vi "checkMotorOverheat.vi"(8 "error in (no error)":errorcluster, 11 "Model in":refnum<class "Model.lvclass">) -> (0 "error out":errorcluster, 3 "Model out":refnum<class "Model.lvclass">)   [LabVIEW 2015]
uses:
  ApplicationElements/Thermocouple/Thermocouple.lvclass
  Model.lvclass
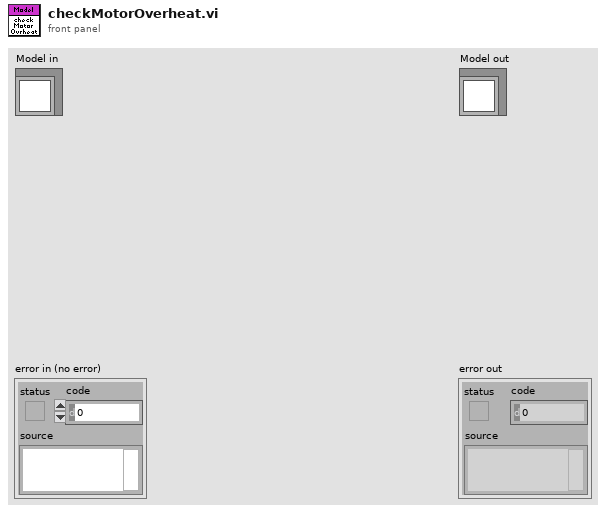
[diagram p1: front panel]
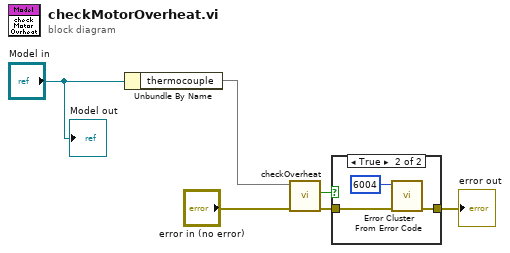
[diagram p0: block diagram]
diagram:
  n1 = Unbundle By Name("Model in") -> ("thermocouple"=w4)
  n2 = call "checkOverheat.vi"("error in (no error)"="error in (no error)", "Thermocouple in"=w4) -> ("error out"=w1:errorcluster, "overtempIsTrue"=w3:bool)  [unwired: 7 in, 1 out]
  n3 = case shown="True" w3 {
    tunnel: [w7 w10] -> w6
    tunnel: w1 -> [w7 w9]
    frame False {
    }
    frame True {
      n4 = call <vilib>:"Error Cluster From Error Code.vi"("error in (no error)"=w9, "error code (0)"=6004) -> ("error out"=w10:errorcluster)  [unwired: 7 in]
    }
  }
  "error out" <- w6
  "Model out" <- "Model in"
